vi "Find all dependencies of vis in memory.vi"(7 "Open FP's of Parents?":bool, 8 "error in":errorcluster, 10 "Include .ctl's":bool, 11 "Include .vi's":bool=TRUE) -> (0 "error out":errorcluster, 1 "Project":string, 2 "Dependencies":T1[](array[typedef]))   [LabVIEW 2010]
doc: "This .vi will list the .vis in memory that are not present in the current project. This is more useful than the project explorer's dependency list, because it does not include code that is present in disabled diagrams (as long as that block diagram is not in memory)."
uses:
  Dependency cluster.ctl
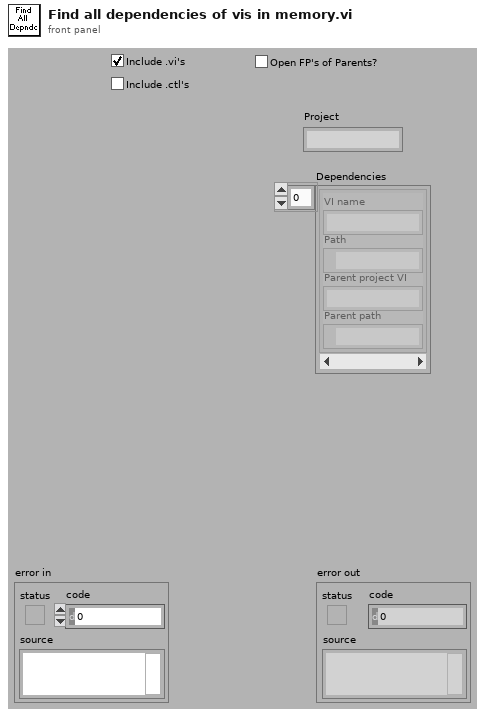
[diagram p1: front panel]
types:
  T1 = typedef "Dependency cluster.ctl" = cluster{"VI name":string, "Path":path, "Parent project VI":string, "Parent path":path}
  T2 = enum32{"Invalid", "Standard", "Closed", "Hidden", "Minimized", "Maximized"}
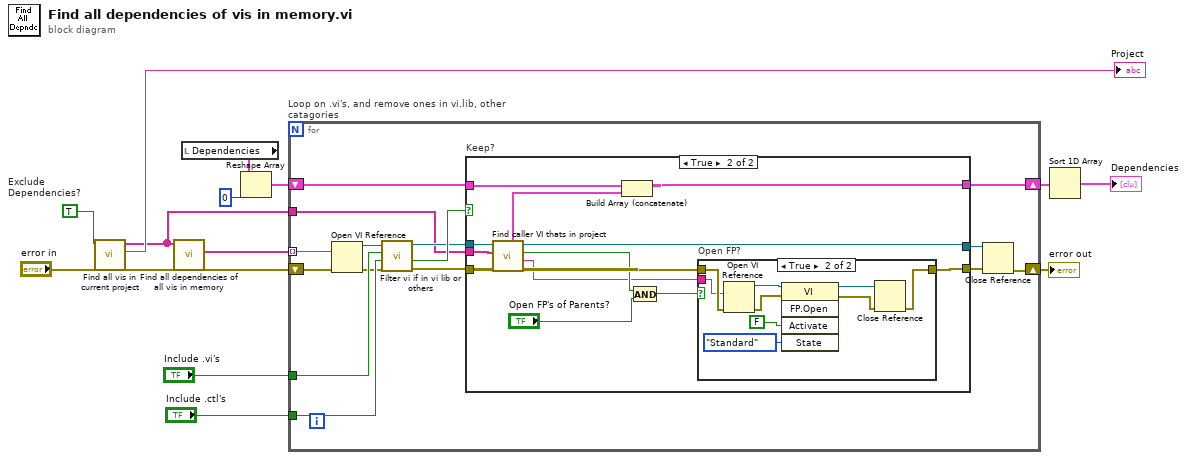
[diagram p0: block diagram]
diagram:
  w15 = TRUE  # Exclude Dependencies?
  n1 = call "Find all vis in current project.vi"("error in"="error in", "ExcludeDependencies?"=w15) -> ("error out"=w14:errorcluster, "Project name"=→"Project":string, "All VIs in .proj"=w3:string[])  [unwired: 3 out]
  n2 = call "Find all dependencies of all vis in memory.vi"("error in"=w14, "All VIs in .proj"=w3) -> ("error out"=w4:errorcluster, "Dependencies"=w5:string[])  [unwired: 4 out]
  n3 = local read "Dependencies"() -> (w13:T1[])
  n4 = Reshape Array(w13, 0 ("dimension size")) -> (w12:T1[])
  n5 = for "Loop on .vi's, and remove ones in vi.lib, other catagories" {
    tunnel: w5 -> [w17] mode=indexing
    shift-right: [w27] -> w8
    shift-left: w4 -> [w18]
    shift-right: [w30] -> w10
    shift-left: w12 -> [w29]
    tunnel: w3 -> [w22]
    tunnel: "Include .vi's" -> [w21]
    tunnel: "Include .ctl's" -> [w20]
    n6 = Open VI Reference(vi path=w17, error in (no error)=w18) -> (vi reference=w16:refnum<vi>, error out=w19:errorcluster)  [unwired: 4 out]
    n7 = call "Filter vi if in vi lib or others.vi"("error in"=w19, "Include .ctl's"=w20, "Include .vi's"=w21, "vi reference in"=w16) -> ("error out"=w26:errorcluster, "Boolean"=w28:bool, "vi reference (dup)"=w25:refnum<vi>)  [unwired: 1 out]
    n8 = case "Keep?" shown="True" w28 {
      tunnel: w29 -> [w33 w46]
      tunnel: [w33 w45] -> w30
      tunnel: w26 -> [w31 w44]
      tunnel: w25 -> [w32 w43]
      tunnel: [w31 w35] -> w24
      tunnel: [w32 w41] -> w23
      tunnel: w22 -> [_ w42]
      frame False {
      }
      frame True {
        n9 = call "Find caller VI thats in project.vi"("error in"=w44, "All VIs in .proj"=w42, "VI Refnum"=w43) -> ("error out"=w37:errorcluster, "Parent Project VI"=w36:string, "Parent found?"=w38:bool, "VI Refnum (dup)"=w41:refnum<vi>, "VI details"=w34:T1)  [unwired: 4 out]
        n10 = Build Array (concatenate)(w46, w34) -> (w45:T1[])
        n11 = And(x=w38, y="Open FP's of Parents?") -> (x .and. y?=w40:bool)
        n12 = case "Open FP?" shown="True" w40 {
          tunnel: w37 -> [w47 w52]
          tunnel: w36 -> [_ w51]
          tunnel: [w47 w50] -> w35
          frame False {
          }
          frame True {
            n13 = Open VI Reference(vi path=w51, error in (no error)=w52) -> (vi reference=w56:refnum<vi>, error out=w55:errorcluster)  [unwired: 4 out]
            n14 = invoke class="VI" method="FP.Open"(reference=w56, error in=w55, "Activate"=FALSE ("Activate?"), "State"=T2."Standard") -> (reference out=w49:refnum<vi>, error out=w48:errorcluster)  [unwired: 1 in, 3 out]
            n15 = Close Reference(reference=w49, error in (no error)=w48) -> (error out=w50:errorcluster)
          }
        }
      }
    }
    n16 = Close Reference(reference=w23, error in (no error)=w24) -> (error out=w27:errorcluster)
  }
  "error out" <- w8
  n17 = Sort 1D Array(array=w10) -> (sorted array=→"Dependencies":T1[])
